vi "read gain subvi.vi"(0 "VISA resource name":refnum<visa-resource-name>="GPIB0::12::INSTR", 1 "write buffer":string="RDA", 2 "bytes to read (1000)":u32=1000, 3 "error in (no error)":errorcluster, 5 "read? (f)":bool=TRUE) -> (4 "bytes read":u32, 6 "VISA resource name out":refnum<visa-resource-name>, 7 "read buffer":string, 8 "result string":string, 9 "error out":errorcluster)   [LabVIEW 2009]
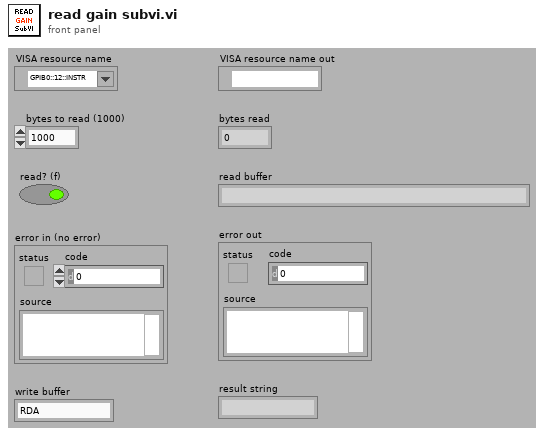
[diagram p1: front panel]
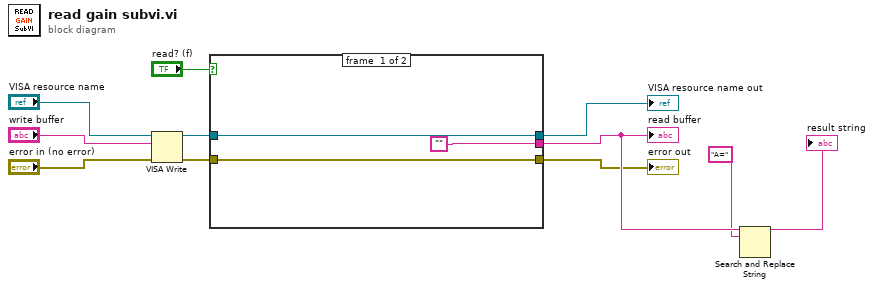
[diagram p0: block diagram]
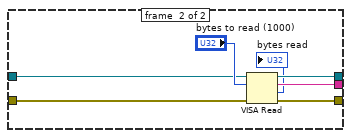
[diagram p2: hidden frame]
diagram:
  n1 = VISA Write(VISA resource name="VISA resource name", write buffer="write buffer", error in (no error)="error in (no error)") -> (VISA resource name out=w6:refnum<visa-resource-name>, error out=w7:errorcluster)  [unwired: 1 out]
  n2 = case shown="True" "read? (f)" {
    tunnel: w7 -> [w13 w15]
    tunnel: [w13 w21] -> w3
    tunnel: [w14 w19] -> w4
    tunnel: w6 -> [w14 w16]
    tunnel: ["" w18] -> w9
    frame #0 {
    }
    frame #1 {
      n3 = VISA Read(VISA resource name=w16, byte count="bytes to read (1000)", error in (no error)=w15) -> (VISA resource name out=w19:refnum<visa-resource-name>, read buffer=w18:string, return count=→"bytes read":u32, error out=w21:errorcluster)
    }
  }
  "error out" <- w3
  "read buffer" <- w9
  "VISA resource name out" <- w4
  n4 = Search and Replace String(input string=w9, search string="A=") -> (result string=→"result string":string)  [unwired: 6 in, 3 out]
